vi "Sequence Init.vi"(8 "error in (no error)":errorcluster, 11 "SimSyA in":refnum<class "SimSyA.lvclass">) -> (0 "error out":errorcluster, 3 "SimSyA out":refnum<class "SimSyA.lvclass">)   [LabVIEW 2014, in "SimSyA.lvlib" / "SimSyA.lvclass"]
uses:
  SimSyA.lvclass
  SimSyA.lvclass/SimSyA.ctl
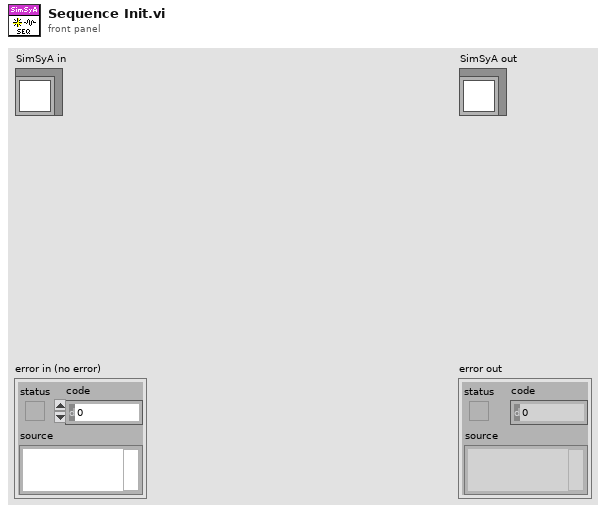
[diagram p1: front panel]
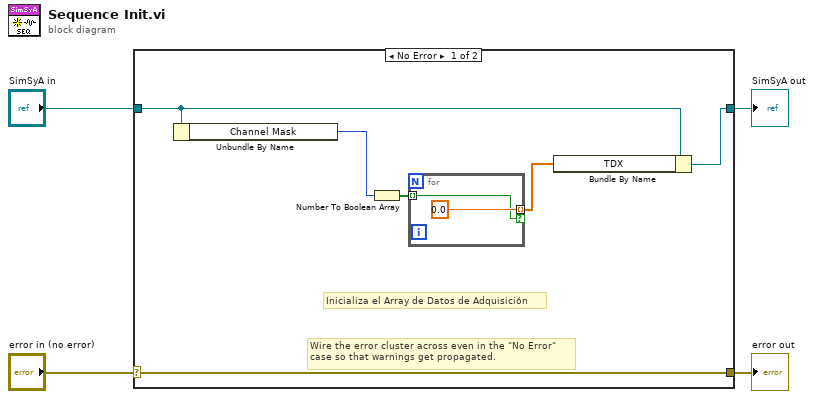
[diagram p0: block diagram]
diagram:
  n1 = case shown="No Error" "error in (no error)" {
    selector: "error in (no error)" -> [w10 w14]
    tunnel: [w10 w14] -> w3
    tunnel: [w9 w13] -> w1
    tunnel: "SimSyA in" -> [w6 w13]
    frame No Error {
      # "Inicializa el Array de Datos de Adquisición"
      # "Wire the error cluster across even in the \"No Error\"\ncase so that warnings get propagated."
      n2 = Unbundle By Name(w6) -> ("Channel Mask"=w5:u64)
      n3 = Number To Boolean Array(number=w5) -> (Boolean array=w8:bool[])
      n4 = for {
        tunnel: w8 -> [w11] mode=indexing
        tunnel: [sgl 0.0] -> w7 mode=indexing if=w11
      }
      n5 = Bundle By Name(cluster=w6, "TDX"=w7) -> (w9:refnum<class "SimSyA.lvclass">)
    }
    frame Error {
    }
  }
  "error out" <- w3
  "SimSyA out" <- w1
